vi "Read Listeners.vi"(8 "error in (no error)":errorcluster, 11 "Trace Controller in":refnum<class "Trace Controller.lvclass">) -> (0 "error out":errorcluster, 2 "Listeners":refnum<class "Message Enqueuer.lvclass">[](array[class]), 3 "Trace Controller out":refnum<class "Trace Controller.lvclass">)   [LabVIEW 2014, in "Robot Actor Framework.lvlib" / "Trace.lvlib" / "Trace Controller.lvclass"]
uses:
  Trace Controller.lvclass
  <vilib>/ActorFramework/Message Enqueuer/Message Enqueuer.lvclass
  Trace Controller.lvclass/Trace Controller.ctl
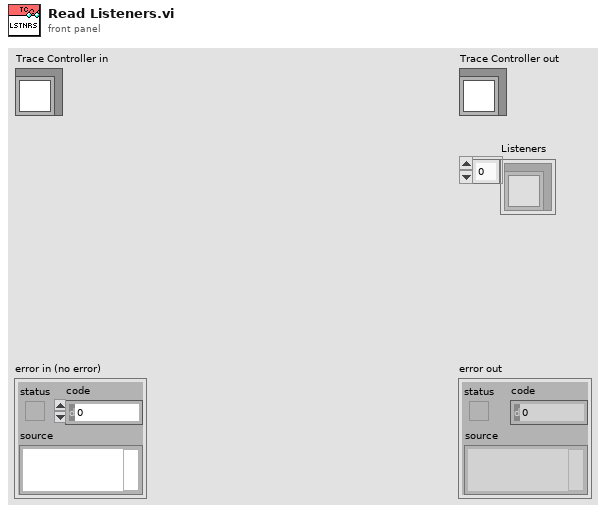
[diagram p1: front panel]
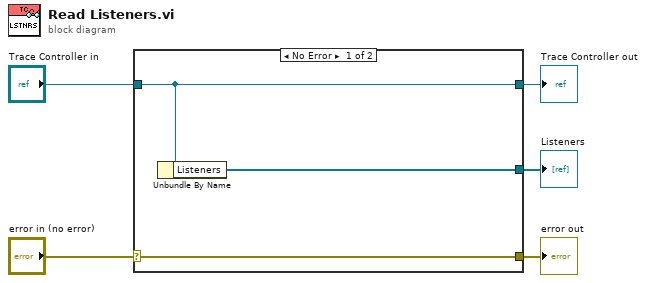
[diagram p0: block diagram]
diagram:
  n1 = case shown="No Error" "error in (no error)" {
    selector: "error in (no error)" -> [w8 w9]
    tunnel: [w8 w9] -> w4
    tunnel: [w7 w10] -> w2
    tunnel: "Trace Controller in" -> [w7 w10]
    tunnel: [w6 _] -> w1
    frame No Error {
      n2 = Unbundle By Name(w7) -> ("Listeners"=w6:refnum<class "Message Enqueuer.lvclass">[])
    }
    frame Error {
    }
  }
  "error out" <- w4
  "Trace Controller out" <- w2
  "Listeners" <- w1
